vi "AlarmTable.vi"(0 "HH值":dbl, 1 "H值":dbl, 2 "L值":dbl, 3 "LL值":dbl, 5 "报警值":string, 6 "单位":string, 7 "报警形式":string, 8 "消除时间":string, 9 "确认时间":string, 10 "报警时间":string, 11 "名称":string) -> (4 "error out":errorcluster caption="错误输出")   [LabVIEW 2012]
panel:
  in  "Command Text":string="INSERT INTO SurroundingDataTable(名称,报警时间,确认时间,消除时间,报警形式,报警值,单位,LL值,L值,H值,HH值) VALUES('名称的位置','报警时间的位置','确认时间的位置','消除时间的位置','报警形式的位置','报警值的位置','单位的位置','LL值的位置','L值的位置','H值的位置','HH值的位置');"
  in  "ConnectionString":string="Provider=Microsoft.ACE.OLEDB.12.0;Data Source= "
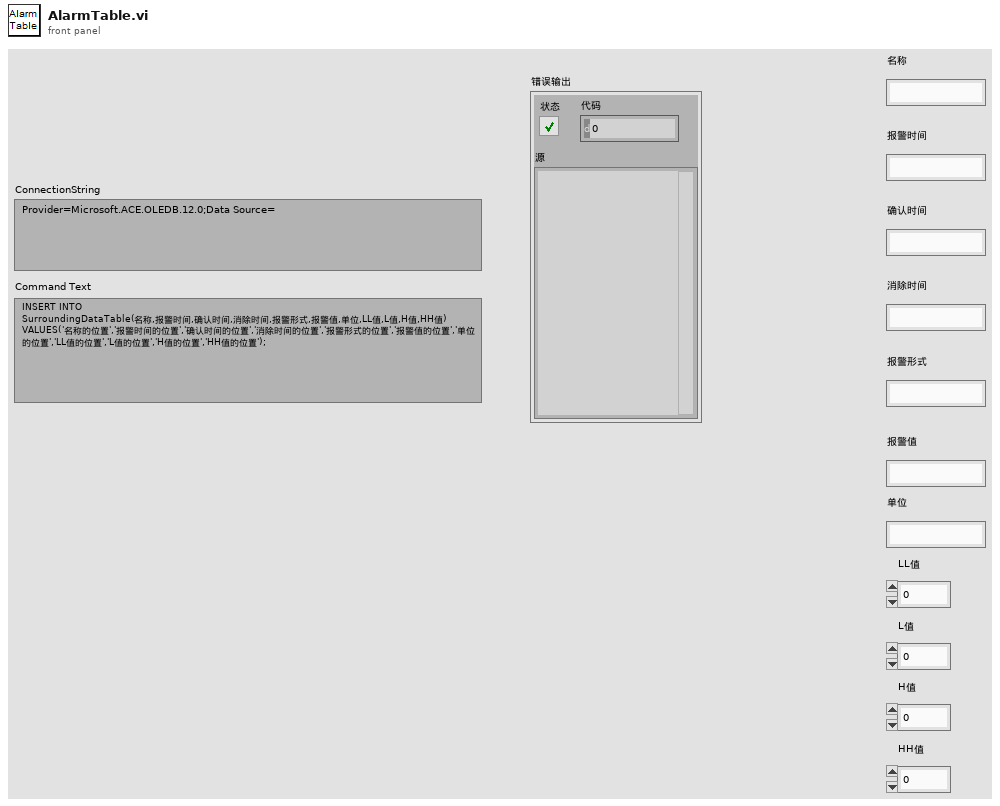
[diagram p1: front panel]
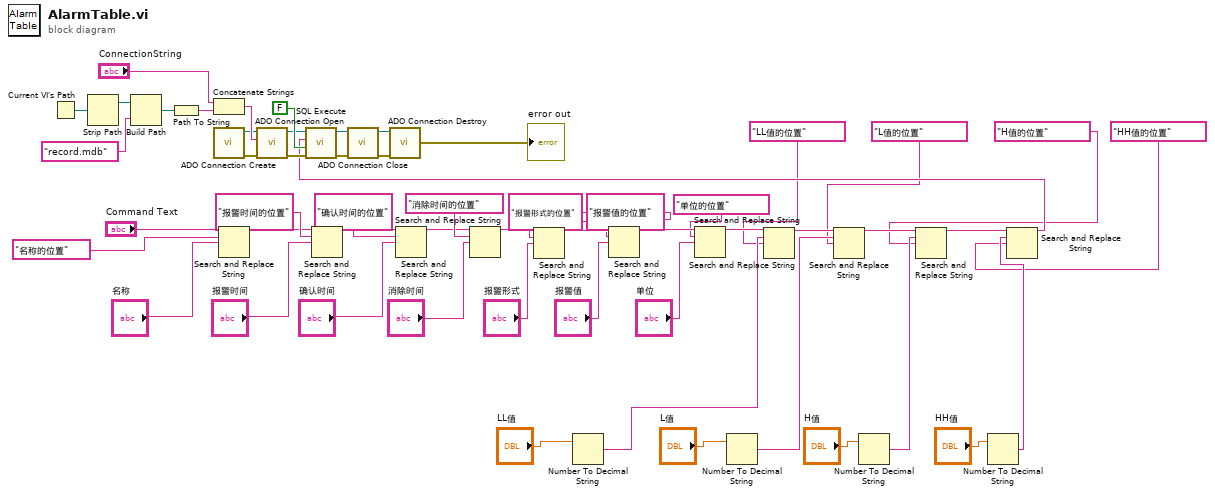
[diagram p0: block diagram]
diagram:
  n1 = Current VI's Path() -> (path=w45:path)
  n2 = Strip Path(path=w45) -> (stripped path=w44:path)  [unwired: 1 out]
  n3 = Build Path(base path=w44, name or relative path="record.mdb") -> (appended path=w47:path)
  n4 = Path To String(path=w47) -> (string=w42:string)
  n5 = Concatenate Strings("ConnectionString", w42) -> (w43:string)
  n6 = call <userlib>:"ADO Connection Create.vi"() -> ("error out"=w35:errorcluster, "ADODB._Connection Out"=w36:refnum<k7>)  [unwired: 10 in]
  n7 = Search and Replace String(input string="Command Text", search string="名称的位置", replace string="名称") -> (result string=w50:string)  [unwired: 5 in, 3 out]
  n8 = call <userlib>:"ADO Connection Open.vi"("error in (no error)"=w35, "ConnectionString"=w43, "ADODB._Connection In"=w36) -> ("error out"=w34:errorcluster, "ADODB._Connection Out"=w37:refnum<k7>)  [unwired: 7 in]
  n9 = Search and Replace String(input string=w50, search string="报警时间的位置", replace string="报警时间") -> (result string=w51:string)  [unwired: 5 in, 3 out]
  n10 = Search and Replace String(input string=w51, search string="确认时间的位置", replace string="确认时间") -> (result string=w52:string)  [unwired: 5 in, 3 out]
  n11 = Search and Replace String(input string=w52, search string="消除时间的位置", replace string="消除时间") -> (result string=w26:string)  [unwired: 5 in, 3 out]
  n12 = Search and Replace String(input string=w26, search string="报警形式的位置", replace string="报警形式") -> (result string=w25:string)  [unwired: 5 in, 3 out]
  n13 = Number To Decimal String(number="LL值") -> (decimal integer string=w12:string)  [unwired: 1 in]
  n14 = Search and Replace String(input string=w25, search string="报警值的位置", replace string="报警值") -> (result string=w24:string)  [unwired: 5 in, 3 out]
  n15 = Search and Replace String(input string=w24, search string="单位的位置", replace string="单位") -> (result string=w17:string)  [unwired: 5 in, 3 out]
  n16 = Number To Decimal String(number="L值") -> (decimal integer string=w11:string)  [unwired: 1 in]
  n17 = Search and Replace String(input string=w17, search string=w12, replace string="LL值的位置") -> (result string=w16:string)  [unwired: 5 in, 3 out]
  n18 = Search and Replace String(input string=w16, search string=w11, replace string="L值的位置") -> (result string=w15:string)  [unwired: 5 in, 3 out]
  n19 = Number To Decimal String(number="H值") -> (decimal integer string=w10:string)  [unwired: 1 in]
  n20 = Search and Replace String(input string=w15, search string=w10, replace string="H值的位置") -> (result string=w14:string)  [unwired: 5 in, 3 out]
  n21 = Number To Decimal String(number="HH值") -> (decimal integer string=w9:string)  [unwired: 1 in]
  n22 = Search and Replace String(input string=w14, search string=w9, replace string="HH值的位置") -> (result string=w13:string)  [unwired: 5 in, 3 out]
  n23 = call <userlib>:"SQL Execute.vi"("error in (no error)"=w34, "Return Data (T)"=FALSE, "Command Text"=w13, "ADODB._Connection In"=w37) -> ("error out"=w33:errorcluster, "ADODB._Connection Out"=w38:refnum<k7>)  [unwired: 4 in, 2 out]
  n24 = call <userlib>:"ADO Connection Close.vi"("error in (no error)"=w33, "ADODB._Connection In"=w38) -> ("error out"=w32:errorcluster, "ADODB._Connection Out"=w39:refnum<k7>)  [unwired: 8 in]
  n25 = call <userlib>:"ADO Connection Destroy.vi"("error in (no error)"=w32, "ADODB._Connection In"=w39) -> ("error out"=→"error out":errorcluster)  [unwired: 9 in]
